vi "TDMS Playback for VST_9-28-2017.vi"(4 "IQ Swap Enabled":bool=TRUE, 6 "pre filter gain":dbl, 7 "channel name (iq/qi)":string="iq", 8 "IQ Rate (S/s)":dbl=25000000.0 format="%#_3p", 9 "Output Power (dBm)":dbl format="%#_3p", 10 "Carrier (Hz)":dbl=3550000000.0 format="%#_3p", 11 "Path":path=path "\\\\tsclient\\X/Shared-Data for Group Users/playBackTestSignals/newSynthTestSignalsDec2017/testRadarSynthPeakPowdBwWithNoise-70.json") -> (0 "error out":errorcluster)   [LabVIEW 2017]
uses:
  <instrlib>/niRFSG/niRFSG.llb/niRFSG Write Arb Waveform (Complex DBL).vi
  <vilib>/FPGAPlugInAG/Dynamic/niLvFpga_Close_Dynamic.vi
  <vilib>/rvi/interface/nirviCloseFPGA/nirviCloseFPGA.xnode
panel:
  out "20 log (scale Factor_Linear)":dbl=-118.76037846648316
  in  "Scale Factor Linear":dbl=1.1934598400763813e-07
  in  "RF:LO Out Enabled":bool
  out "RF:LO Out Power (dBm)":dbl=-0.06505490226659383
  in  "RF:External Gain (dB)":dbl
  in  "RF:Peak Power Adjustment (dB)":dbl
  out "RF:Peak Envelope Power (dBm) =\nPeak Power Adjustment + Output Power":dbl=-5.0
  out "RF:Upconverter:Gain (dB)":dbl=-9.678101652264932
  out "samples":u32=1090503665
  out "number of pending reads 1":u32=8
  out "empty elements":u32=134217728
  out "dma fullness":u32=63200
  out "number of pending reads 2":u32=1
  out "# of elements in host buffer avail for writing":u32=65536
  out "peak fullness":u32
  out "fullness":u32=65536
  out "Completion Loop":i32=86113
  out "fpga peak":u32(slide)=176 scale=-1.0..65536.0
  in  "Monitor Buffer Fullness":bool=TRUE
  out "file peak":u32(slide)=1 scale=0.0..8.0
  out "host peak":u32(slide)=768 scale=-1.0..134217728.0
  out "File Read Buffer Fullness":u32(slide)=1 scale=0.0..8.0
  out "Playback Progress":i32(slide)=535 scale=-1.0..357.0
  out "DMA Host Buffer Emptiness":u32(slide) scale=-1.0..134217728.0
  out "DMA FPGA Buffer Emptiness":u32(slide)=464 scale=-1.0..65536.0
  out "Underflow Detected":bool
  in  "stop button":bool
  in  "Read Block Size (MB)":u32=32 caption="Chunk Size (S)" format="%.0f MB"
  in  "chunks":u32=16 caption="DMA Host Buffer Depth (Blocks)" format="%.0p"
  in  "VST Resource":string="VST"
  # "Config"
  # "Status"
  # "File"
  # "Current"
  # "10/11/2017: +8.57dBm gave -7.23dBm output of the highest peak \n==> Compensate and used Output Power of +8.57+0.24=\n+8.8 dBM to get -7dBm"
  # "Peak"
  # "Current"
  # "Peak"
  # "10/19/2017: +8.8dBm gave -6.44dBm output of the highest peak \n==> Compensate and used Output Power of +8.8-0.47=\n+8.33 dBM to get -7dBm"
  # "RF"
  # "Current"
  # "Peak"
  # "10/19/2017: AutoCal \n==> +8.33 dBm gave -7.22dBm output of the highest peak \n==> Compensate and used Output Power of +8.33+0.22=\n+8.55 dBM to get -7dBm"
  # "Before any other signal processing. \nReduce it to prevent overflow in the AWG interpolation filters. \nSaturates at 7 dB."
  # "After filtering. \nAdjust the output power while keeping the analog path fixed."
  # "Compensate for any Attenuation/Amplification \nbetween Output and DUT"
  # "Refers to PAPR, only used in PEAK Power type.\nIt adds up to Output Power."
  # "20log(1.1534E-6)=  -118.76 dBW\n-118.76 dBW + Correction Factor = -16 dBW \nCorrection Factor = 104.6 dBW"
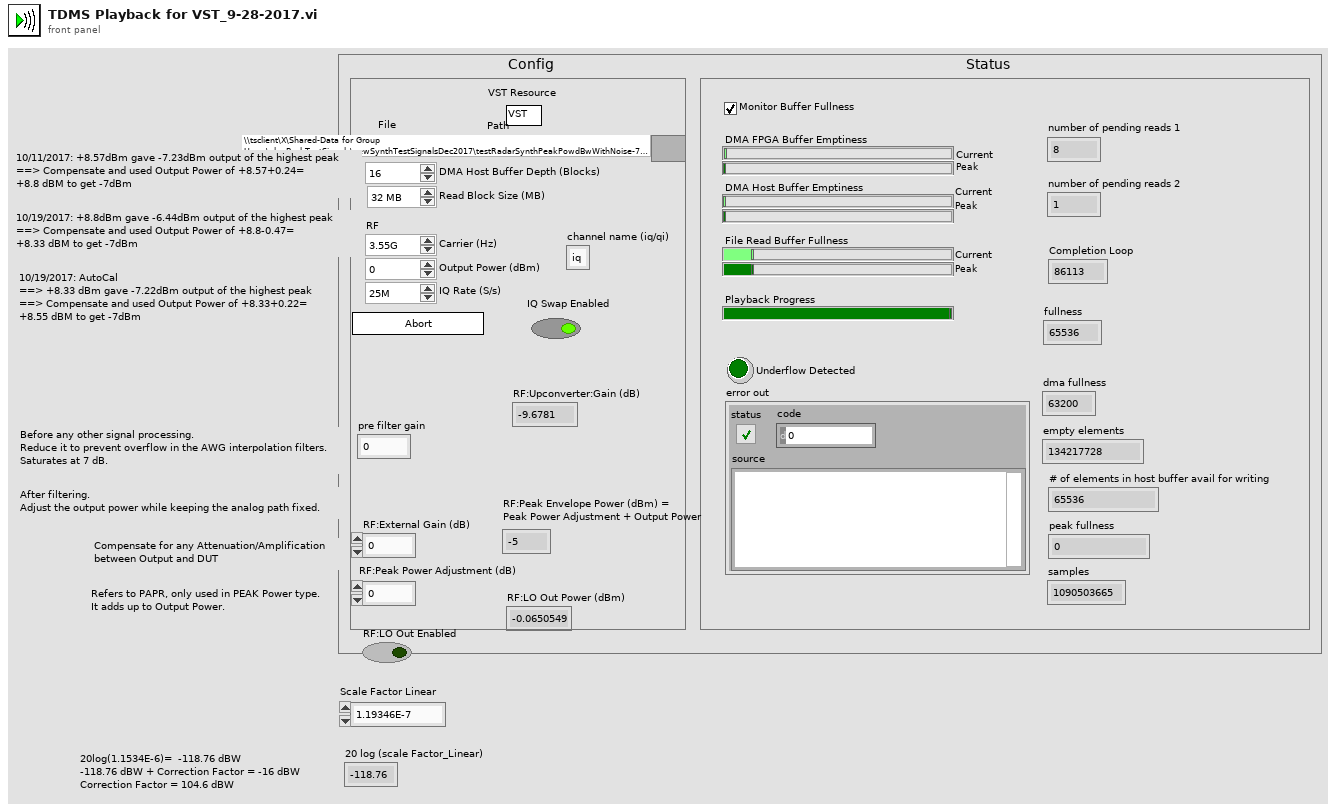
[diagram p1: front panel]
types:
  T1 = enum16{"open", "open or create", "create or replace", "create", "open (read-only)"}
  T2 = cluster{"underflow":bool, "underflows":u32, "samples":u32}
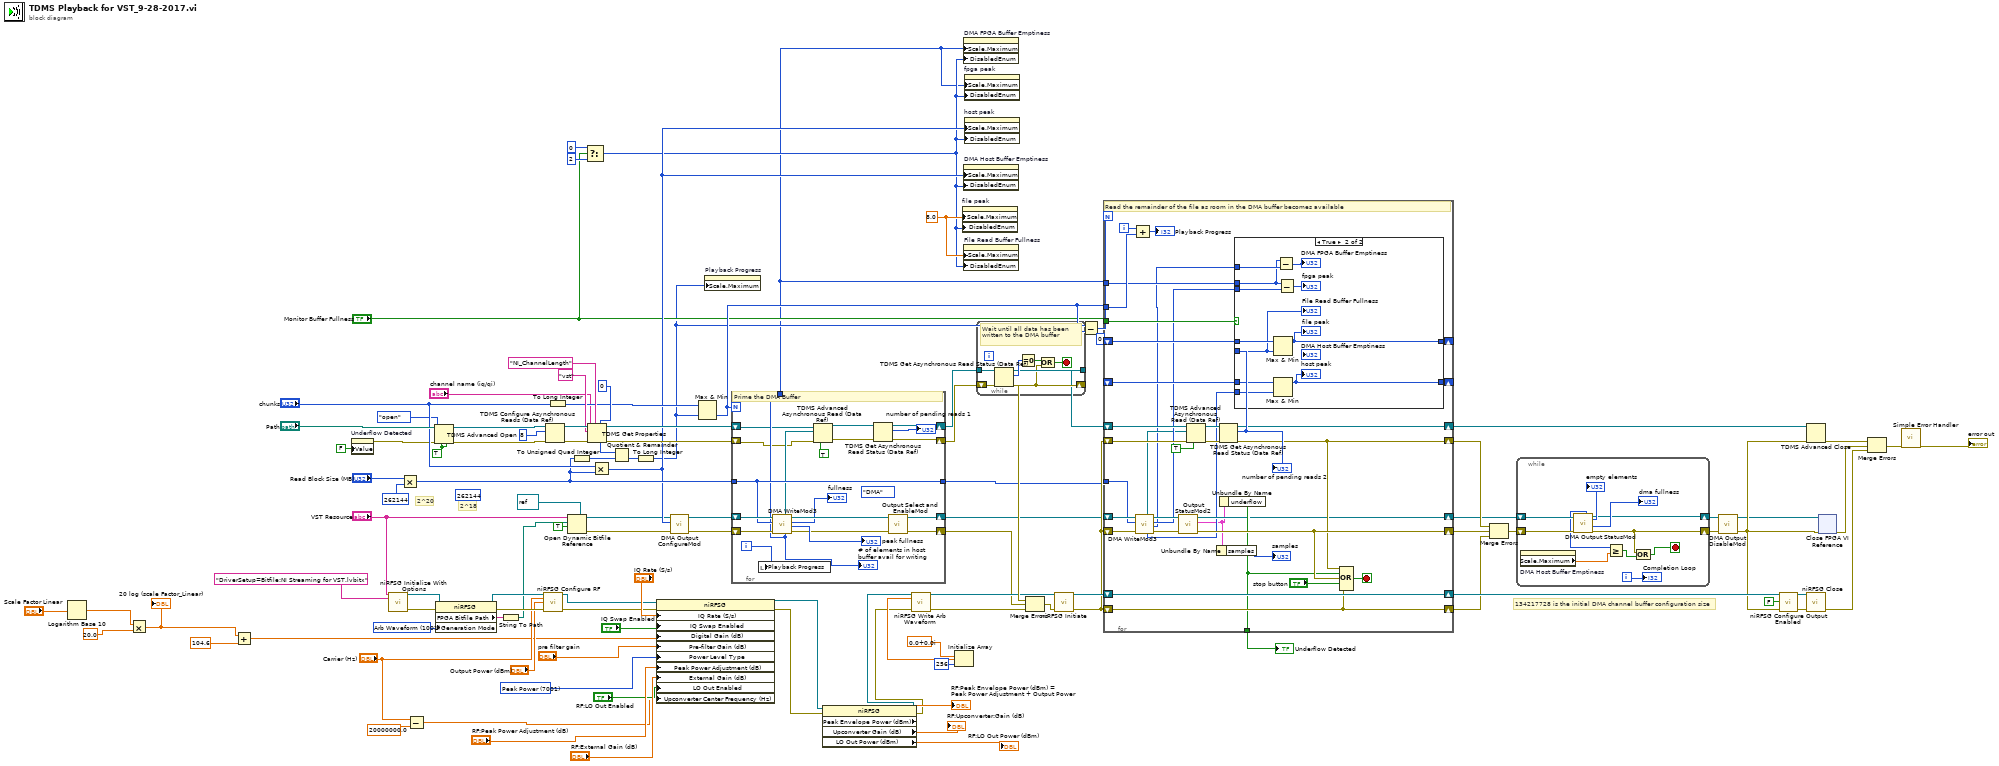
[diagram p0: block diagram]
diagram:
  w24 = 7001 items=["Average Power"=7000, "Peak Power"=7001] ("RF:Power Level Type")
  (unwired) u32 262144 ("y")
  w50 = 8.0 ("Scale.Range:Maximum")
  w12 = TRUE ("disable buffering? (T)")
  w105 = 1001 items=["CW"=1000, "Arb Waveform"=1001, "Script"=1002] ("Arb:Generation Mode")
  # "134217728 is the initial DMA channel buffer configuration size"
  # "2^20"
  # "2^18"
  n1 = Logarithm Base 10(1:"Scale Factor Linear") -> (0:w6:dbl)
  n2 = Multiply(x=w6, y=20.0) -> (x*y=w5:dbl)
  "20 log (scale Factor_Linear)" <- w5
  n3 = Add(x=w5, y=104.6) -> (x+y=w1:dbl)
  n4 = property on="Underflow Detected" class="Bool (strict)"("Value"=FALSE ("Underflow Detected")) -> (error out=w48:errorcluster)  [unwired: 2 in, 1 out]
  n5 = call <instrlib>:"niRFSG Initialize With Options.vi"("resource name"="VST Resource", "option string"="DriverSetup=Bitfile:NI Streaming for VST.lvbitx") -> ("instrument handle"=w110:refnum<k15>, "error out"=w111:errorcluster)  [unwired: 12 in]
  n6 = Multiply(x="Read Block Size (MB)", y=u32 262144) -> (x*y=w58:u32)
  n7 = Subtract(x="Carrier (Hz)", y=20000000.0) -> (x-y=w7:dbl)
  n8 = TDMS Advanced Open(4:w12, 6:w12, 8:w48, 10:T1."open" ("operation (0:open)"), 11:"Path") -> (0:w101:errorcluster, 3:w100:refnum<k34>)  [unwired: 1 out]
  n9 = property class="niRFSG"(reference=w110, error in=w111, "Generation Mode"=w105) -> (reference out=w108:refnum<k15>, error out=w109:errorcluster, "FPGA Bitfile Path"=w107:string)
  n10 = String To Path(string=w107) -> (path=w36:path)
  n11 = call <instrlib>:"niRFSG Configure RF.vi"("instrument handle"=w108, "frequency (Hz)"="Carrier (Hz)", "power level (dBm)"="Output Power (dBm)", "error in"=w109) -> ("instrument handle out"=w23:refnum<k15>, "error out"=w22:errorcluster)  [unwired: 10 in]
  n12 = TDMS Configure Asynchronous Reads (Data Ref)(8:w101, 10:u32 8 ("max asynchronous reads (4)"), 11:w100) -> (0:w89:errorcluster, 3:w90:refnum<k34>)  [unwired: 2 in]
  n13 = To Long Integer(number="chunks") -> (32bit integer=w83:i32)
  n14 = Open Dynamic Bitfile Reference(0:"VST Resource", 1:w36, 2:TRUE ("Run When Loaded"), 4:refnum<k20> refnum ("Type")) -> (5:w27:refnum<k20>, 8:w26:errorcluster)  [unwired: 1 in]
  n15 = To Unsigned Quad Integer(1:w58) -> (0:w61:u64)
  n16 = Select(t=0, s="Monitor Buffer Fullness", f=2) -> (s? t:f=w42:i32)
  n17 = TDMS Get Properties(5:u64 0, 7:"NI_ChannelLength" ("property name"), 8:w89, 9:"channel name (iq/qi)", 10:"vst" ("group name"), 11:w90) -> (0:w87:errorcluster, 3:w88:refnum<k34>, 4:w66:u64)  [unwired: 3 out]
  n18 = Multiply(x="chunks", y=w58) -> (x*y=w56:u32)
  n19 = Quotient & Remainder(x=w66, y=w61) -> (floor(x/y)=w65:u64)  [unwired: 1 out]
  n20 = To Long Integer(number=w65) -> (32bit integer=w51:i32)
  n21 = property class="niRFSG"(reference=w23, error in=w22, "IQ Rate (S/s)"="IQ Rate (S/s)", "IQ Swap Enabled"="IQ Swap Enabled", "Digital Gain (dB)"=w1, "Pre-filter Gain (dB)"="pre filter gain", "Power Level Type"=w24, "Peak Power Adjustment (dB)"="RF:Peak Power Adjustment (dB)", "External Gain (dB)"="RF:External Gain (dB)", "LO Out Enabled"="RF:LO Out Enabled", "Upconverter Center Frequency (Hz)"=w7) -> (reference out=w19:refnum<k15>, error out=w17:errorcluster)
  n22 = call "DMA Output ConfigureMod.vi"("error in (no error)"=w26, "depth"=w56, "Refnum in"=w27) -> ("error out"=w44:errorcluster, "Refnum out"=w43:refnum<k20>)  [unwired: 7 in]
  n23 = Max & Min(x=w83, y=w51) -> (min(x,y)=w60:i32)  [unwired: 1 out]
  n24 = property on="Playback Progress" class="Slide (strict)"("Scale.Maximum"=w51) -> ()  [unwired: 2 in, 2 out]
  n25 = for {
    N: w60 -> [_]
    shift-right: [w117] -> w97
    shift-left: w87 -> [w113]
    shift-right: [w120] -> w47
    shift-left: w44 -> [w129]
    shift-right: [w116] -> w98
    shift-left: w88 -> [w114]
    shift-right: [w128] -> w45
    shift-left: w43 -> [w130]
    tunnel: w58 -> [w127]
    tunnel: [w127] -> w35
    tunnel: [w125] -> w41
    i -> [w126]
    (unwired) enum16{"none", "DMA", "local", "P2P", "DIO"}."DMA" ("stream select")
    # "Prime the DMA Buffer"
    n26 = local write "Playback Progress"(w126) -> ()
    n27 = call "DMA WriteMod3.vi"("error in (no error)"=w129, "number of elements"=w127, "Refnum in"=w130) -> ("error out"=w120:errorcluster, "peak fullness"=→"peak fullness":u32, "fullness"=→"fullness":u32, "Refnum out"=w128:refnum<k20>, "empty elements remaining"=w125:u32, "Write Region Reference"=w124:refnum<data-value>)  [unwired: 3 in]
    "# of elements in host buffer avail for writing" <- w125
    n28 = TDMS Advanced Asynchronous Read (Data Ref)(6:TRUE ("auto delete reference? (T)"), 8:w113, 10:w124, 11:w114) -> (0:w118:errorcluster, 3:w119:refnum<k34>)  [unwired: 1 out]
    n29 = TDMS Get Asynchronous Read Status (Data Ref)(8:w118, 11:w119) -> (0:w117:errorcluster, 2:→"number of pending reads 1":u32, 3:w116:refnum<k34>)
  }
  n30 = property class="niRFSG"(reference=w19, error in=w17) -> (reference out=w18:refnum<k15>, error out=w16:errorcluster, "Peak Envelope Power (dBm)"=→"RF:Peak Envelope Power (dBm) =\nPeak Power Adjustment + Output Power":dbl, "Upconverter Gain (dB)"=→"RF:Upconverter:Gain (dB)":dbl, "LO Out Power (dBm)"=→"RF:LO Out Power (dBm)":dbl)
  n31 = call "Output Select and EnableMod.vi"("error in (no error)"=w47, "Refnum in"=w45) -> ("error out"=w46:errorcluster, "Refnum out"=w38:refnum<k20>)  [unwired: 8 in]
  n32 = Initialize Array(cdb 0.0+0.0i ("element"), 256 ("dimension size")) -> (w32:cdb[])
  n33 = call-poly <instrlib>:"niRFSG Write Arb Waveform.vi"("instrument handle"=w18, "waveform data"=w32, "error in"=w16) -> ("instrument handle out"=w81:refnum<k15>, "error out"=w80:errorcluster)  [unwired: 11 in]
  n34 = property on="file peak" class="Slide (strict)"("Scale.Maximum"=w50, "DisabledEnum"=w42) -> ()  [unwired: 2 in, 2 out]
  n35 = property on="DMA FPGA Buffer Emptiness" class="Slide (strict)"("Scale.Maximum"=w41, "DisabledEnum"=w42) -> ()  [unwired: 2 in, 2 out]
  n36 = property on="DMA Host Buffer Emptiness" class="Slide (strict)"("Scale.Maximum"=w56, "DisabledEnum"=w42) -> ()  [unwired: 2 in, 2 out]
  n37 = property on="File Read Buffer Fullness" class="Slide (strict)"("Scale.Maximum"=w50, "DisabledEnum"=w42) -> ()  [unwired: 2 in, 2 out]
  n38 = property on="fpga peak" class="Slide (strict)"("Scale.Maximum"=w41, "DisabledEnum"=w42) -> ()  [unwired: 2 in, 2 out]
  n39 = property on="host peak" class="Slide (strict)"("Scale.Maximum"=w56, "DisabledEnum"=w42) -> ()  [unwired: 2 in, 2 out]
  n40 = while {
    tunnel: w98 -> [w136]
    shift-right: [w132] -> w94
    shift-left: w97 -> [w137]
    tunnel: [w134] -> w93
    stop <- w133 stop-if-true
    # "Wait until all data has been written to the DMA buffer"
    n41 = TDMS Get Asynchronous Read Status (Data Ref)(8:w137, 11:w136) -> (0:w132:errorcluster, 2:w135:u32, 3:w134:refnum<k34>)
    n42 = Equal To 0?(x=w135) -> (x = 0?=w131:bool)
    n43 = Or(x=w131, y=w132) -> (x .or. y?=w133:bool)
  }
  n44 = Merge Errors(w94, w46, w80) -> (w96:errorcluster)
  n45 = call <instrlib>:"niRFSG Initiate.vi"("instrument handle"=w81, "error in"=w96) -> ("instrument handle out"=w95:refnum<k15>, "error out"=w82:errorcluster)  [unwired: 12 in]
  n46 = Subtract(x=w51, y=w60) -> (x-y=w59:i32)
  n47 = for {
    N: w59 -> [_]
    shift-right: [w171] -> w69
    shift-left: w82 -> [w171]
    shift-right: [w151] -> w70
    shift-left: w82 -> [w158]
    shift-right: [w154] -> w71
    shift-left: w82 -> [w159]
    shift-right: [w150] -> w91
    shift-left: w93 -> [w157]
    shift-right: [w172] -> w77
    shift-left: w95 -> [w172]
    tunnel: w60 -> [w168]
    tunnel: w35 -> [w144]
    tunnel: [w148] -> w57
    shift-right: [w164] -> _
    shift-left: u32 0 -> [w163]
    shift-right: [w162] -> _
    shift-left: _ -> [w161]
    tunnel: "Monitor Buffer Fullness" -> [w160]
    tunnel: w41 -> [w147]
    shift-right: [w143] -> w37
    shift-left: w38 -> [w145]
    i -> [w167]
    stop <- w169 stop-if-true
    # "Read the remainder of the file as room in the DMA buffer becomes available"
    n48 = Add(x=w167, y=w168) -> (x+y=→"Playback Progress":i32)
    n49 = call "DMA WriteMod3.vi"("error in (no error)"=w159, "number of elements"=w144, "Refnum in"=w145) -> ("error out"=w155:errorcluster, "peak fullness"=w140:u32, "fullness"=w149:u32, "Refnum out"=w156:refnum<k20>, "empty elements remaining"=w142:u32, "Write Region Reference"=w141:refnum<data-value>)  [unwired: 3 in]
    n50 = call "Output StatusMod2.vi"("error in (no error)"=w155, "Refnum in"=w156) -> ("error out"=w154:errorcluster, "status"=w139:T2, "Refnum out"=w143:refnum<k20>)  [unwired: 7 in]
    n51 = TDMS Advanced Asynchronous Read (Data Ref)(6:TRUE ("auto delete reference? (T)"), 8:w158, 10:w141, 11:w157) -> (0:w153:errorcluster, 3:w152:refnum<k34>)  [unwired: 1 out]
    n52 = Unbundle By Name(w139) -> ("samples"=→"samples":u32)
    n53 = TDMS Get Asynchronous Read Status (Data Ref)(8:w153, 11:w152) -> (0:w151:errorcluster, 2:w165:u32, 3:w150:refnum<k34>)
    "number of pending reads 2" <- w165
    n54 = Unbundle By Name(w139) -> ("underflow"=w148:bool)
    n55 = case shown="True" w160 {
      tunnel: w165 -> [_ w182]
      tunnel: [_ w180] -> w164
      tunnel: w163 -> [_ w183]
      tunnel: [_ w179] -> w162
      tunnel: w161 -> [_ w181]
      tunnel: w140 -> [_ w175]
      tunnel: w149 -> [_ w177]
      tunnel: w142 -> [_ w178]
      tunnel: w147 -> [_ w174]
      frame False {
      }
      frame True {
        n56 = Max & Min(x=w183, y=w182) -> (max(x,y)=w180:u32)  [unwired: 1 out]
        "file peak" <- w180
        n57 = Max & Min(x=w181, y=w178) -> (max(x,y)=w179:u32)  [unwired: 1 out]
        "host peak" <- w179
        n58 = Subtract(x=w174, y=w175) -> (x-y=→"DMA FPGA Buffer Emptiness":u32)
        n59 = Subtract(x=w174, y=w177) -> (x-y=→"fpga peak":u32)
        "File Read Buffer Fullness" <- w182
      }
    }
    n60 = Compound Arithmetic op=OR(w151, w148, w154, "stop button", w171) -> (w169:bool)
  }
  "Underflow Detected" <- w57
  n61 = Merge Errors(w70, w71, w69) -> (w92:errorcluster)
  n62 = while {
    shift-right: [w189] -> w79
    shift-left: w92 -> [w193]
    shift-right: [w184] -> w78
    shift-left: w37 -> [w192]
    i -> [w191]
    stop <- w190 stop-if-true
    n63 = property on="DMA Host Buffer Emptiness" class="Slide (strict)"() -> ("Scale.Maximum"=w185:dbl)  [unwired: 2 in, 2 out]
    n64 = call "DMA Output StatusMod.vi"("error in (no error)"=w193, "Refnum in"=w192) -> ("error out"=w189:errorcluster, "dma fullness"=→"dma fullness":u32, "Refnum out"=w184:refnum<k20>, "empty elements"=w186:u32)  [unwired: 5 in, 1 out]
    "empty elements" <- w186
    n65 = Greater Or Equal?(x=w186, y=w185) -> (x >= y?=w188:bool)
    n66 = Compound Arithmetic op=OR(w189, w188) -> (w190:bool)
    "Completion Loop" <- w191
  }
  n67 = call "DMA Output DisableMod.vi"("error in (no error)"=w79, "Refnum in"=w78) -> ("error out"=w29:errorcluster, "Refnum out"=w28:refnum<k20>)  [unwired: 8 in]
  n68 = call <instrlib>:"niRFSG Configure Output Enabled.vi"("instrument handle"=w77, "output enabled"=FALSE, "error in"=w29) -> ("instrument handle out"=w75:refnum<k15>, "error out"=w76:errorcluster)  [unwired: 11 in]
  n69 = TDMS Advanced Close(8:w29, 11:w91) -> (0:w64:errorcluster)  [unwired: 2 in, 1 out]
  n70 = call <instrlib>:"niRFSG Close.vi"("instrument handle"=w75, "error in"=w76) -> ("error out"=w62:errorcluster)  [unwired: 13 in]
  n71 = xnode "Close FPGA VI Reference"("FPGA VI Reference In"=w28, "error in"=w29) -> ("error out"=w63:errorcluster)
  n72 = Merge Errors(w64, w63, w62) -> (w30:errorcluster)
  "error out" <- w30
  n73 = call <vilib>:"Simple Error Handler.vi"("error in (no error)"=w30) -> ()  [unwired: 4 in, 5 out]
